vi "Get Register.vi"(11 "jettl in":refnum<class "jettl.lvclass">) -> (2 "Register":refnum<event-registration>)   [LabVIEW 2021, in "jettl.lvlib" / "jettl.lvclass"]
uses:
  jettl.lvclass
  Msg Strategy/Msg Strategy.lvclass
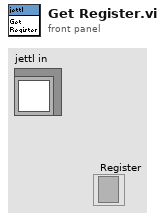
[diagram p1: front panel]
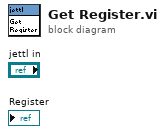
[diagram p0: block diagram]
diagram:
